vi "Serialize.vi"(8 "error in (no error)":errorcluster, 11 "DiagramConverter in":refnum<class "DiagramConverter.lvclass">) -> (0 "error out":errorcluster, 2 "JSON":string, 3 "DiagramConverter out":refnum<class "DiagramConverter.lvclass">)   [LabVIEW 2017, in "DiagramConverter.lvclass"]
uses:
  DiagramConverter.lvclass
panel:
  out "Dependency Names":string[](array[string])
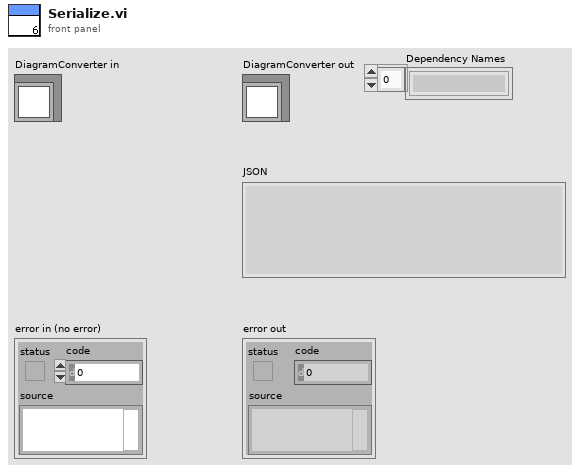
[diagram p1: front panel]
types:
  T1 = typedef "imagedata.ctl" = cluster{"image type":i32, "image depth":i32, "image":u8[], "mask":u8[], "colors":u32[], "Rectangle":cluster{"left":i16, "top":i16, "right":i16, "bottom":i16}}
  T2 = enum8{"No dynamic dispatch VIs", "Include nearest implementation", "Include all overrides"}
  T3 = typedef "LVRectTypeDef.ctl" = cluster{"Left":i16, "Top":i16, "Right":i16, "Bottom":i16}
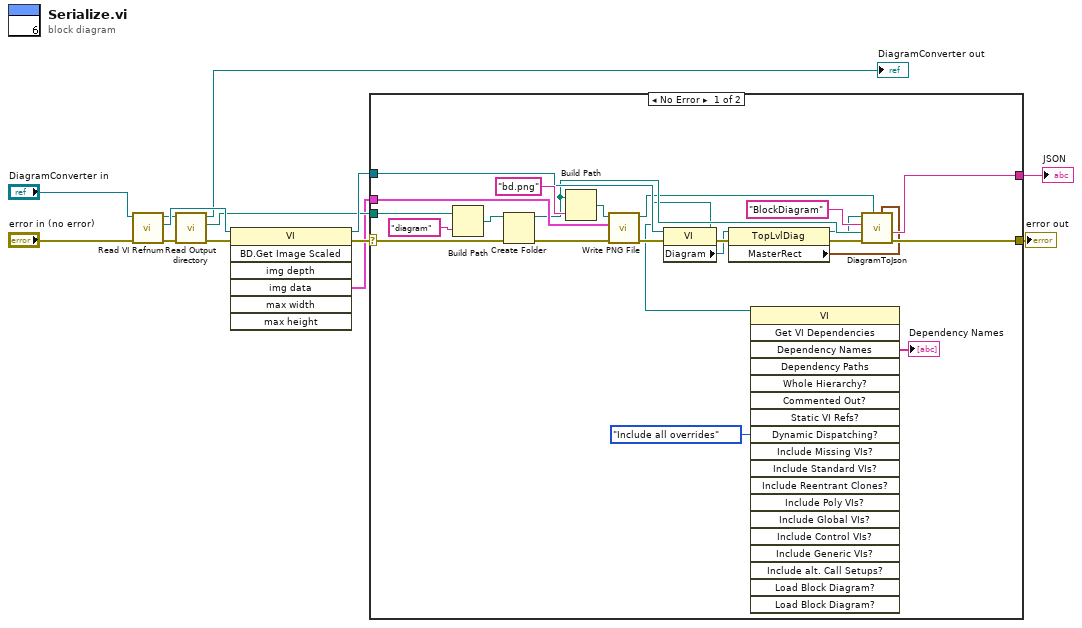
[diagram p0: block diagram]
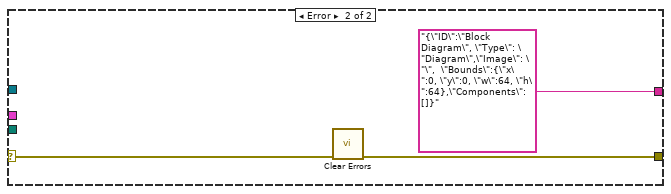
[diagram p2: hidden frame]
diagram:
  n1 = call-dynamic "Read VI Refnum.vi"("error in (no error)"="error in (no error)", "VIObjectConverter in"="DiagramConverter in") -> ("error out"=w2:errorcluster, "VI Refnum"=w10:refnum<vi>, "VIObjectConverter out"=w9:refnum<class "DiagramConverter.lvclass">)  [unwired: 7 in]
  n2 = call-dynamic "Read Output directory.vi"("error in (no error)"=w2, "GObjectConverterBase in"=w9) -> ("error out"=w1:errorcluster, "Output directory"=w7:path, "GObjectConverterBase out"=→"DiagramConverter out":refnum<class "DiagramConverter.lvclass">)  [unwired: 7 in]
  n3 = invoke class="VI" method="BD.Get Image Scaled"(reference=w10, error in=w1) -> (reference out=w12:refnum<vi>, error out=w13:errorcluster, "img data"=w6:T1)  [unwired: 5 in, 4 out]
  n4 = case shown="No Error" w13 {
    selector: w13 -> [w23 w38]
    tunnel: w7 -> [w26 _]
    tunnel: w12 -> [w22 _]
    tunnel: [w36 "{\"ID\":\"Block Diagram\", \"Type\": \"Diagram\",\"Image\": \"\",  \"Bounds\":{\"x\":0, \"y\":0, \"w\":64, \"h\":64},\"Components\": []}" ("JSON (out)")] -> w3
    tunnel: [w34 w37] -> w4
    tunnel: w6 -> [w25 _]
    frame No Error {
      n5 = Build Path(base path=w26, name or relative path="diagram" ("string")) -> (appended path=w32:path)
      n6 = Create Folder(path (use dialog)=w32, error in=w23) -> (created path=w20:path, error out=w24:errorcluster)  [unwired: 1 in, 1 out]
      n7 = Build Path(base path=w20, name or relative path="bd.png" ("string")) -> (appended path=w33:path)
      n8 = call <vilib>:"Write PNG File.vi"("error in (no error)"=w24, "image data"=w25, "path to PNG file"=w33) -> ("error out"=w29:errorcluster, "path"=w19:path)  [unwired: 7 in]
      n9 = property class="VI"(reference=w22, error in=w29) -> (reference out=w16:refnum<vi>, error out=w31:errorcluster, "Diagram"=w30:refnum<vi>)
      n10 = property class="TopLvlDiag"(reference=w30, error in=w31) -> (reference out=w18:refnum<vi>, error out=w17:errorcluster, "MasterRect"=w21:T3)
      n11 = invoke class="VI" method="Get VI Dependencies"(reference=w16, "Dynamic Dispatching?"=T2."Include all overrides") -> ("Dependency Names"=→"Dependency Names":string[])  [unwired: 17 in, 18 out]
      n12 = call "DiagramToJson.vi"("Owner Bounds"=w21, "Image Path"=w19, "error in (no error)"=w17, "Current Path"=w20, "ID"="BlockDiagram", "GObj in"=w18) -> ("error out"=w34:errorcluster, "JSON (out)"=w36:string)  [unwired: 3 in, 1 out]
    }
    frame Error {
      n13 = call <vilib>:"Clear Errors.vi"("error in (no error)"=w38) -> ("error out"=w37:errorcluster)  [unwired: 5 in, 1 out]
    }
  }
  "error out" <- w4
  "JSON" <- w3
